vi "GraphStopOrExit.vi"   [LabVIEW 2018]
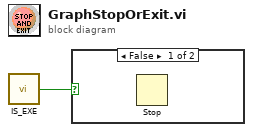
[diagram p0: block diagram]
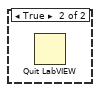
[diagram p2: hidden frame]
diagram:
  n1 = call "IS_EXE.vi"() -> ("1 - EXE"=w1:bool)  [unwired: 3 in, 2 out]
  n2 = case shown="False" w1 {
    frame False {
      n3 = Stop() -> ()  [unwired: 1 in]
    }
    frame True {
      n4 = Quit LabVIEW() -> ()  [unwired: 1 in]
    }
  }
